vi "Append Content to Current Page.vi"(8 "error in (no error)":errorcluster {"code" format="Error %.0f"}, 10 "Content":string, 11 "VIDoc Printer - Confluence In":refnum<class "VIDoc Printer - Confluence.lvclass">) -> (0 "error out":errorcluster {"code" format="Error %.0f"}, 3 "VIDoc Printer - Confluence Out":refnum<class "VIDoc Printer - Confluence.lvclass">)   [LabVIEW 2023, in "VIDoc Printer - Confluence.lvlib" / "VIDoc Printer - Confluence.lvclass"]
uses:
  VIDoc Printer - Confluence.lvclass
  VIDoc Printer - Confluence.lvclass/VIDoc Printer - Confluence.ctl
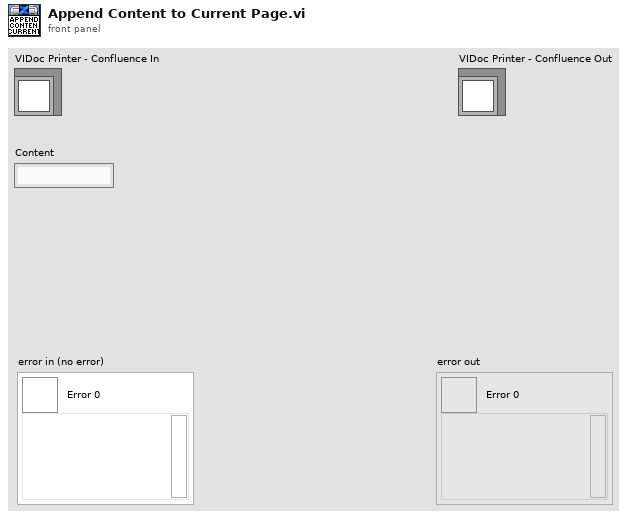
[diagram p1: front panel]
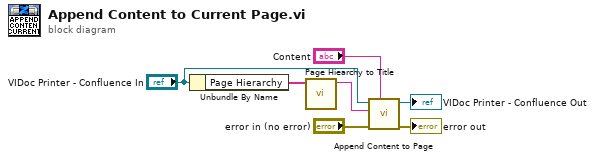
[diagram p0: block diagram]
diagram:
  n1 = Unbundle By Name("VIDoc Printer - Confluence In") -> ("Page Hierarchy"=w7:string[])
  n2 = call "Page Hiearchy to Title.vi"("Page Hierarchy"=w7) -> ("Page Title"=w1:string)  [unwired: 10 in]
  n3 = call "Append Content to Page.vi"("Page Content"="Content", "error in (no error)"="error in (no error)", "Page Title"=w1, "VIDoc Printer - Confluence In"="VIDoc Printer - Confluence In") -> ("error out"=→"error out":errorcluster, "VIDoc Printer - Confluence Out"=→"VIDoc Printer - Confluence Out":refnum<class "VIDoc Printer - Confluence.lvclass">)  [unwired: 6 in]
